vi "m1m3_getEvent_ForceActuatorDataRejection.vi"(8 "error in (no error)":errorcluster, 11 "logevent_ForceActuatorDataRejection_Ctl":T1) -> (0 "error out":errorcluster, 2 "function return":i32, 3 "logevent_ForceActuatorDataRejection_Ctl out":T1)   [LabVIEW 2016, in "SALLV_m1m3.lvlib"]
doc: "int m1m3_shm_getEvent_ForceActuatorDataRejectionLV(m1m3_logevent_ForceActuatorDataRejectionLV *logevent_ForceActuatorDataRejection_Ctl );"
uses:
  SALLV_m1m3.lvlib
  DataTypes/logevent_ForceActuatorDataRejection.ctl
  SALLV_m1m3.so
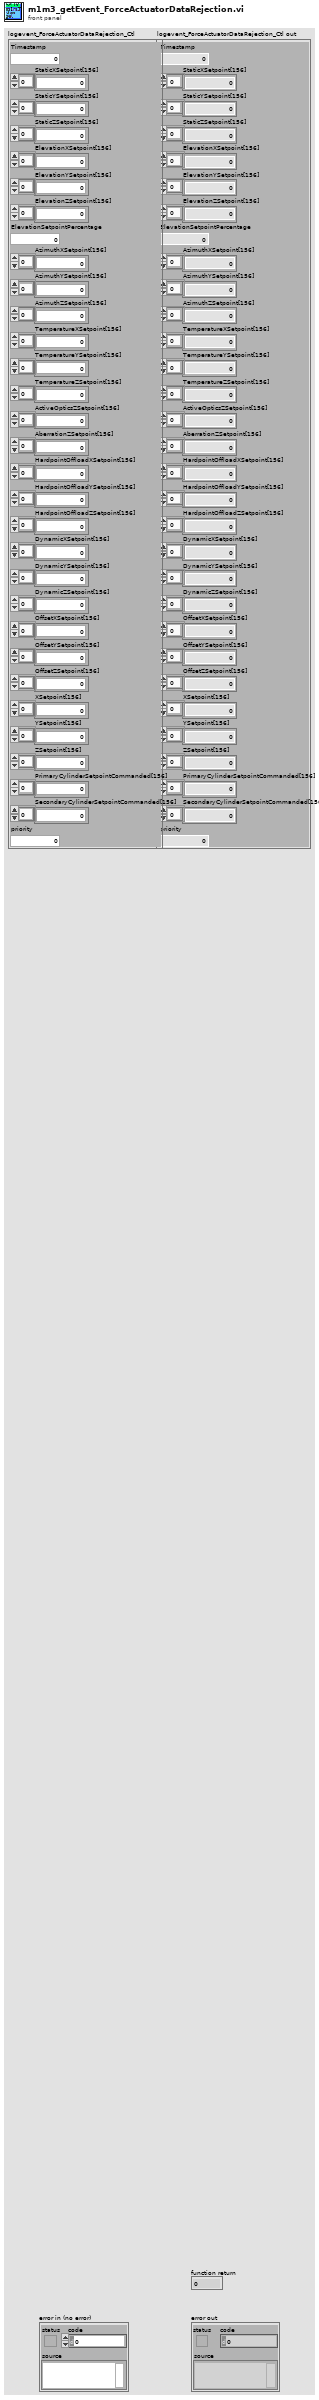
[diagram p1: front panel]
types:
  T1 = typedef "SALLV_m1m3.lvlib/logevent_ForceActuatorDataRejection.ctl" = cluster{"Timestamp":dbl, "StaticXSetpoint[156]":dbl[], "StaticYSetpoint[156]":dbl[], "StaticZSetpoint[156]":dbl[], "ElevationXSetpoint[156]":dbl[], "ElevationYSetpoint[156]":dbl[], "ElevationZSetpoint[156]":dbl[], "ElevationSetpointPercentage":dbl, "AzimuthXSetpoint[156]":dbl[], "AzimuthYSetpoint[156]":dbl[], "AzimuthZSetpoint[156]":dbl[], "TemperatureXSetpoint[156]":dbl[], "TemperatureYSetpoint[156]":dbl[], "TemperatureZSetpoint[156]":dbl[], "ActiveOpticsZSetpoint[156]":dbl[], "AberrationZSetpoint[156]":dbl[], "HardpointOffloadXSetpoint[156]":dbl[], "HardpointOffloadYSetpoint[156]":dbl[], "HardpointOffloadZSetpoint[156]":dbl[], "DynamicXSetpoint[156]":dbl[], "DynamicYSetpoint[156]":dbl[], "DynamicZSetpoint[156]":dbl[], "OffsetXSetpoint[156]":dbl[], "OffsetYSetpoint[156]":dbl[], "OffsetZSetpoint[156]":dbl[], "XSetpoint[156]":dbl[], "YSetpoint[156]":dbl[], "ZSetpoint[156]":dbl[], "PrimaryCylinderSetpointCommanded[156]":i32[], "SecondaryCylinderSetpointCommanded[156]":i32[], "priority":i32}
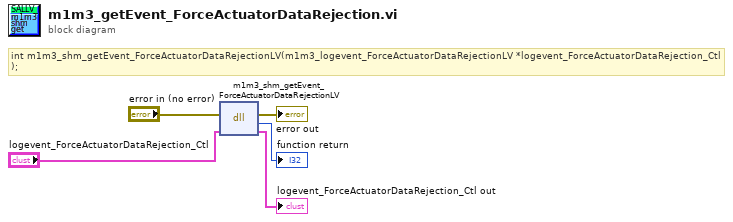
[diagram p0: block diagram]
diagram:
  # "int m1m3_shm_getEvent_ForceActuatorDataRejectionLV(m1m3_logevent_ForceActuatorDataRejectionLV *logevent_ForceActuatorDataRejection_Ctl );"
  n1 = dll-call lib="opt/CODE/SALLV_m1m3/SALLV_m1m3.*" fn="m1m3_shm_getEvent_ForceActuatorDataRejectionLV"(error in="error in (no error)", "logevent_ForceActuatorDataRejection_Ctl"="logevent_ForceActuatorDataRejection_Ctl") -> (error out=→"error out":errorcluster, →"function return":i32, "logevent_ForceActuatorDataRejection_Ctl"=→"logevent_ForceActuatorDataRejection_Ctl out":T1)  [unwired: 2 in, 1 out]
